vi "ParseSysexFirmwareResponse.vi"(8 "error in":errorcluster={"status"=FALSE, "code"=1073676294, "source"="VISA Read in FirmataClient.lvlib:TxRx.vi->Example.vi"}, 11 "Sysex Message":u8[](array[numeric])=[240, 121, 2, 5, 83, 0, 116, 0, 97, 0, 110, 0, 100, 0, 97, 0, 114, 0, 100, 0, 70, 0, 105, 0, 114, 0, 109, 0, 97, 0, 116, 0, 97, 0, 46, 0, 105, 0, 110, 0, 111, 0, 247] format="%x") -> (0 "error out":errorcluster={"status"=FALSE, "code"=1073676294, "source"="VISA Read in FirmataClient.lvlib:TxRx.vi->Example.vi"}, 1 "IsValidSysex":bool=TRUE, 2 "FirmataFirmwareVersion":string="v2.5", 3 "FirmataFirmwareName":string="StandardFirmata.ino")   [LabVIEW 2020]
doc: "Parse a message according to the Firmata Protocol Requirements. \n- https://github.com/firmata/protocol\n- https://github.com/firmata/protocol/blob/master/protocol.md"
uses:
  Controls/FirmataProtocolConstants.ctl
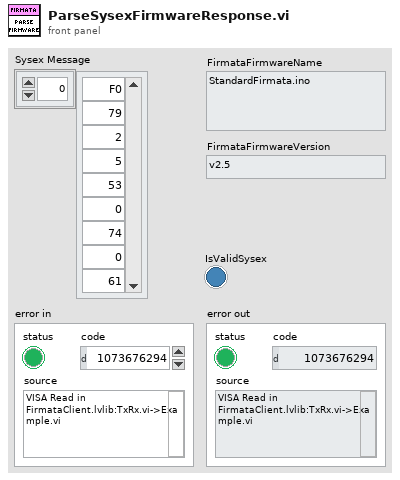
[diagram p1: front panel]
types:
  T1 = typedef "FirmataProtocolConstants.ctl" = u16
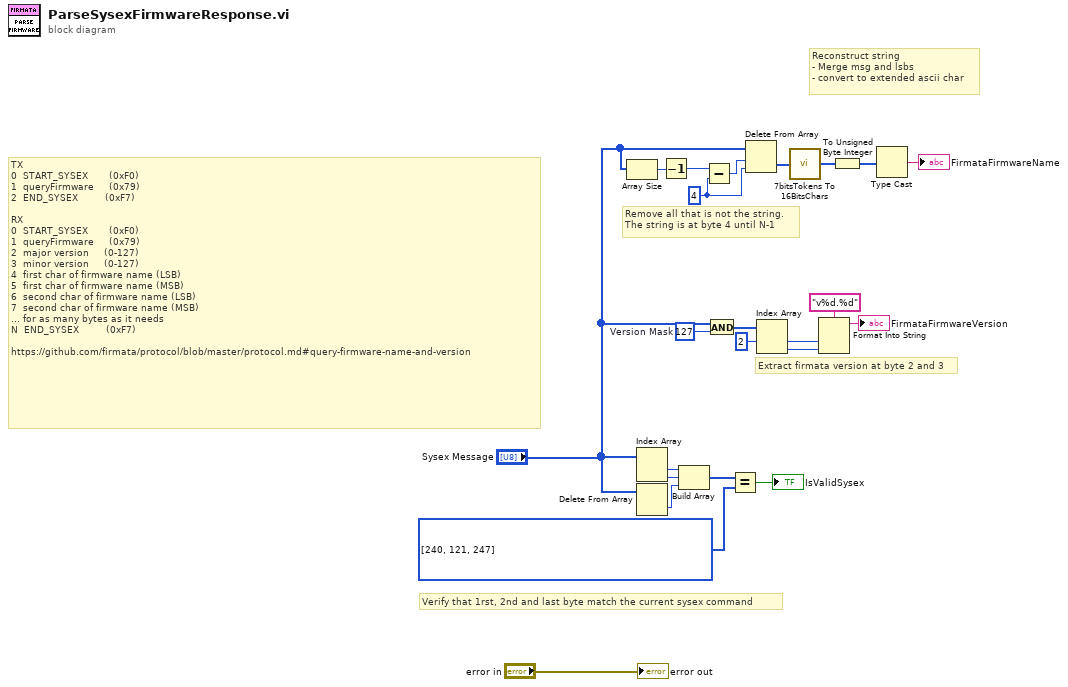
[diagram p0: block diagram]
diagram:
  w5 = T1[] [240, 121, 247] items=["ANALOG_IO_MESSAGE"=224, "DIGITAL_IO_MESSAGE"=144, "REPORT_ANALOG_PIN"=192, "REPORT_DIGITAL_PORT"=208, "START_SYSEX"=240, "END_SYSEX"=247, "SET_PIN_MODE"=244, "SET_DIGITAL_PIN_VALUE"=245, "PROTOCOL_VERSION"=249, "SYSTEM_RESET"=255, "SYSEX.EXTENDED_ID"=0, "SYSEX.RESERVED_USER_COMMANDs"=1, "SYSEX.ANALOG_MAPPING_QUERY"=105, "SYSEX.ANALOG_MAPPING_RESPONSE"=106, "SYSEX.CAPABILITY_QUERY"=107, "SYSEX.CAPABILITY_RESPONSE"=108, "SYSEX.PIN_STATE_QUERY"=109, "SYSEX.PIN_STATE_RESPONSE"=110, "SYSEX.REPORT_FIRMWARE"=121, "SYSEX.EXTENDED_ANALOG"=111, "SYSEX.STRING_DATA"=113, "SYSEX.REALTIME"=127, "SYSEX.NON_REALTIME"=126, "SYSEX.SAMPLING_INTERVAL"=122, "FEATURES.SYSEX.I2C_READ_WRITE"=118, "FEATURES.SYSEX.I2C_REPLY"=119, "FEATURES.SYSEX.I2C_CONFIG"=120]
  w9 = u8 127  # Version Mask
  w16 = 4 ("index")
  # "Reconstruct string\n- Merge msg and lsbs\n- convert to extended ascii char"
  # "Remove all that is not the string. \nThe string is at byte 4 until N-1"
  # "Extract firmata version at byte 2 and 3"
  # "Verify that 1rst, 2nd and last byte match the current sysex command"
  # "TX\n0  START_SYSEX       (0xF0)\n1  queryFirmware     (0x79)\n2  END_SYSEX         (0xF7)\n\nRX\n0  START_SYSEX       (0xF0)\n1  queryFirmware     (0x79)\n2  major version     (0-127)\n3  minor version     (0-127)\n4  first char of firmware name (LSB)\n5  first char of firmware name (MSB)\n6  second char of firmware name (LSB)\n7  second char of firmware name (MSB)\n... for as many bytes as it needs\nN  END_SYSEX         (0xF7)\n\nhttps://github.com/firmata/protocol/blob/master/protocol.md#query-firmware-name-and-version"
  n1 = Array Size(array="Sysex Message") -> (size(s)=w18:i32)
  n2 = Index Array(array="Sysex Message") -> (element #1=w23:u8, element #2=w21:u8)  [unwired: 2 in]
  n3 = Delete From Array(array="Sysex Message") -> (deleted portion=w22:u8)  [unwired: 2 in, 1 out]
  n4 = Decrement(x=w18) -> (x-1=w17:i32)
  n5 = Build Array(w23, w21, w22) -> (w20:u8[])
  n6 = Subtract(x=w17, y=w16) -> (x-y=w15:i32)
  n7 = And(x="Sysex Message", y=w9) -> (x .and. y?=w8:u8[])
  n8 = Equal?(x=w20, y=w5) -> (x = y?=→"IsValidSysex":bool)
  n9 = Delete From Array(array="Sysex Message", length=w15, index=w16) -> (deleted portion=w4:u8[])  [unwired: 1 out]
  n10 = Index Array(array=w8, index #1=2 ("index")) -> (element #1=w13:u8, element #2=w12:u8)  [unwired: 1 in]
  n11 = call "7bitsTokens To 16BitsChars.vi"("Bytes In"=w4) -> ("Words Out"=w2:u16[])
  n12 = Format Into String(format string="v%d.%d", w13, w12) -> (resulting string=→"FirmataFirmwareVersion":string)  [unwired: 2 in, 1 out]
  n13 = To Unsigned Byte Integer(number=w2) -> (unsigned 8bit integer=w1:u8[])
  n14 = Type Cast(x=w1) -> (*(type *) &x=→"FirmataFirmwareName":string)  [unwired: 1 in]
  "error out" <- "error in"
